vi "XY Graph With Motion Indicator.vi"() -> ()   [LabVIEW 2021]
uses:
  <vilib>/Platform/TimedLoop/XDataNode/timing_clust.ctl
  <vilib>/Platform/TimedLoop/XDataNode/nitl_modes.ctl
  <vilib>/Platform/TimedLoop/XDataNode/wakeup.ctl
  <vilib>/platform/TimedLoop/XDataNode/XDataNode.xnode
  <vilib>/Platform/TimedLoop/XDataNode/XDNodeRunTimeDep.lvlib
  <vilib>/Analysis/NI_AALBase.lvlib
panel:
  out "output cluster":cluster{dbl[], dbl[]}
  out "XY Graph":cluster{"sine wave":dbl[], "sine wave":dbl[]}[](graph)
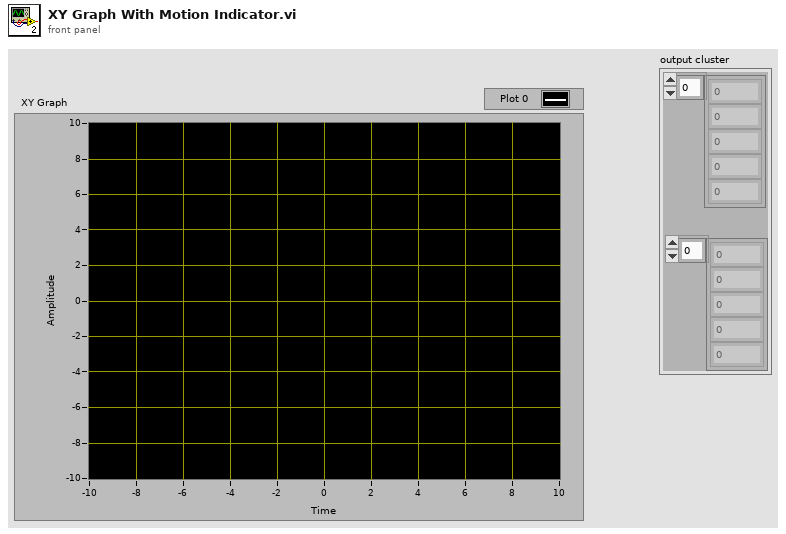
[diagram p1: front panel]
types:
  T1 = typedef "XDNodeRunTimeDep.lvlib/timing_clust.ctl" = cluster{"Expected End [f-1]":u64, "Actual End [f-1]":u64, "Finished Late? [f-1]":bool, "Expected End [i-1]":u64, "Actual End [i-1]":u64, "Finished Late? [i-1]":bool, "Expected Start [i]":u64, "Actual Start [i]":u64, "Expected Start [f]":u64, "Actual Start [f]":u64, "Source Name":string, "Structure Name":string, "Period":i64, "Deadline":i64, "Offset":i64, "Start":i64, "Priority":i32, "Timeout":i32, "Mode":T2, "Wakeup Reason":T3, "Error":errorcluster, "Source Type":string, "Secondary Source Type":string, "Global End Time":u64, "Global Start Time":u64, "Frame Duration":u64, "Iteration Duration":u64, "Assigned CPU":i32, "I/O Scan Engine Mode":u32}
  T2 = typedef "XDNodeRunTimeDep.lvlib/nitl_modes.ctl" = enum32{"No Change", "Process missed periods, maintain original phase", "Discard missed periods, maintain original phase", "Process missed periods, ignore original phase", "Discard missed periods, ignore original phase"}
  T3 = typedef "XDNodeRunTimeDep.lvlib/wakeup.ctl" = enum32{"Normal", "Aborted", "Asynchronous wakeup", "Timing source error", "Timed loop error", "Timeout"}
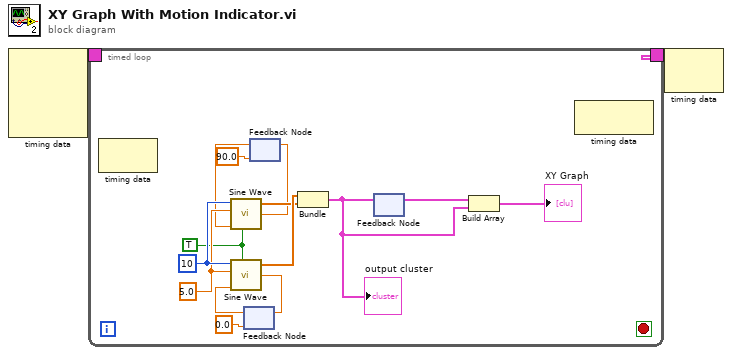
[diagram p0: block diagram]
diagram:
  n1 = node-c288() -> (w2:T1)  [unwired: 4 in]
  n2 = timed-loop {
    timing: w2 -> [_]
    timing-out: [_] -> w1
    stop <- _ stop-if-true
    w12 = TRUE ("reset phase")
    w14 = 5.0 ("amplitude")
    w15 = 10 ("samples")
    n3 = node-c288() -> ()  [unwired: 1 in, 1 out]
    n4 = feedback #1(0.0 ("phase out")) -> (w6:dbl)
    n5 = call <vilib>:"Sine Wave.vi"("samples"=w15, "amplitude"=w14, "phase in"=w6, "reset phase"=w12) -> ("sine wave"=w16:dbl[], "phase out"=w7:dbl)  [unwired: 1 in, 1 out]
    n6 = feedback-in #1(w7) -> ()
    n7 = feedback #2(90.0 ("phase out")) -> (w9:dbl)
    n8 = call <vilib>:"Sine Wave.vi"("samples"=w15, "amplitude"=w14, "phase in"=w9, "reset phase"=w12) -> ("sine wave"=w13:dbl[], "phase out"=w10:dbl)  [unwired: 1 in, 1 out]
    n9 = feedback-in #2(w10) -> ()
    n10 = Bundle("sine wave"=w16, "sine wave"=w13) -> (w4:cluster{"sine wave":dbl[], "sine wave":dbl[]})  [unwired: 1 in]
    "output cluster" <- w4
    n11 = feedback-in #3(w4) -> ()
    n12 = feedback #3() -> (w5:cluster{"sine wave":dbl[], "sine wave":dbl[]})  [unwired: 1 in]
    n13 = Build Array(w5, w4) -> (→"XY Graph":cluster{"sine wave":dbl[], "sine wave":dbl[]}[])
    n14 = node-c288() -> ()  [unwired: 1 in, 1 out]
  }
  n15 = node-c288(w1) -> ()  [unwired: 1 out]
